vi "tag to string.vi"(8 "error in":errorcluster, 11 "tag descriptor in":refnum<class "data bus tag description.lvclass">) -> (0 "error out":errorcluster, 2 "tag string":string, 3 "tag descriptor out":refnum<class "data bus tag description.lvclass">)   [LabVIEW 2013, in "data bus tag description.lvclass"]
uses:
  data bus tag description.lvclass
  data bus tag description.lvclass/data bus tag description.ctl
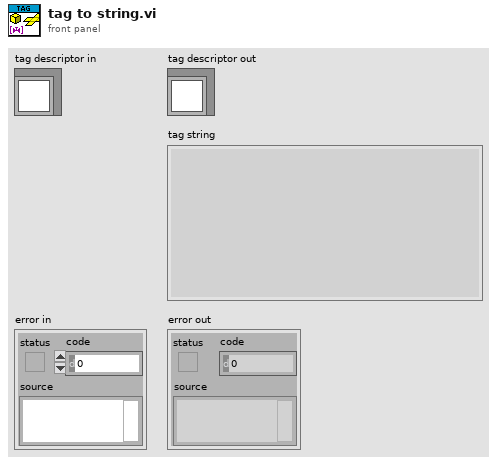
[diagram p1: front panel]
types:
  T1 = cluster{"name":string, "type":string, "default":string, "metadata":string}
  T2 = typedef "data bus tag description.lvclass/Data Type.ctl" = enum16{"Double", "I64", "Boolean", "Array of Double", "Array of I64", "Variant"}
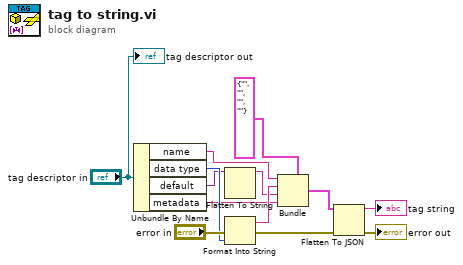
[diagram p0: block diagram]
diagram:
  n1 = Unbundle By Name("tag descriptor in") -> ("name"=w6:string, "data type"=w7:T2, "default"=w1:variant, "metadata"=w4:string)
  n2 = Flatten To String(anything=w1) -> (data string=w2:string)  [unwired: 3 in, 2 out]
  n3 = Format Into String(error in="error in", w7) -> (resulting string=w5:string, error out=w3:errorcluster)  [unwired: 2 in]
  n4 = Bundle(cluster=T1 {"name"="", "type"="", "default"="", "metadata"=""} ("flat tag"), "name"=w6, "type"=w5, "default"=w2, "metadata"=w4) -> (w11:T1)
  n5 = Flatten To JSON(anything=w11, error in (no error)=w3) -> (JSON string=→"tag string":string, 11:→"error out":errorcluster)  [unwired: 1 in]
  "tag descriptor out" <- "tag descriptor in"
